vi "S4 Tool Initial.vi"(8 "error in (no error)":errorcluster) -> (0 "error constant":errorcluster, 3 "S4 InitialStatus":bool)   [LabVIEW 2019]
uses:
  Ctrl/StationCmdSelect.ctl
  Ctrl/Auto Inspection Station Name2.ctl
  Ctrl/Auto Inspection Data Name.ctl
  Global/Process Global.vi
  LineScan/LineScan.lvclass
  LLB/Commonly VI.lvlib
panel:
  out "ToolStringOut_Init":string
  out "Initial_ChkSum":string
  out "Initial receive 2":string
  in  "Numeric 3":i32
  out "Act Step":i32
  out "Numeric":dbl
  out "subarray":string[](array[string])
  out "retry次數":string[](array[string])
  out "CurrentCmd":string
  out "Retry":i32
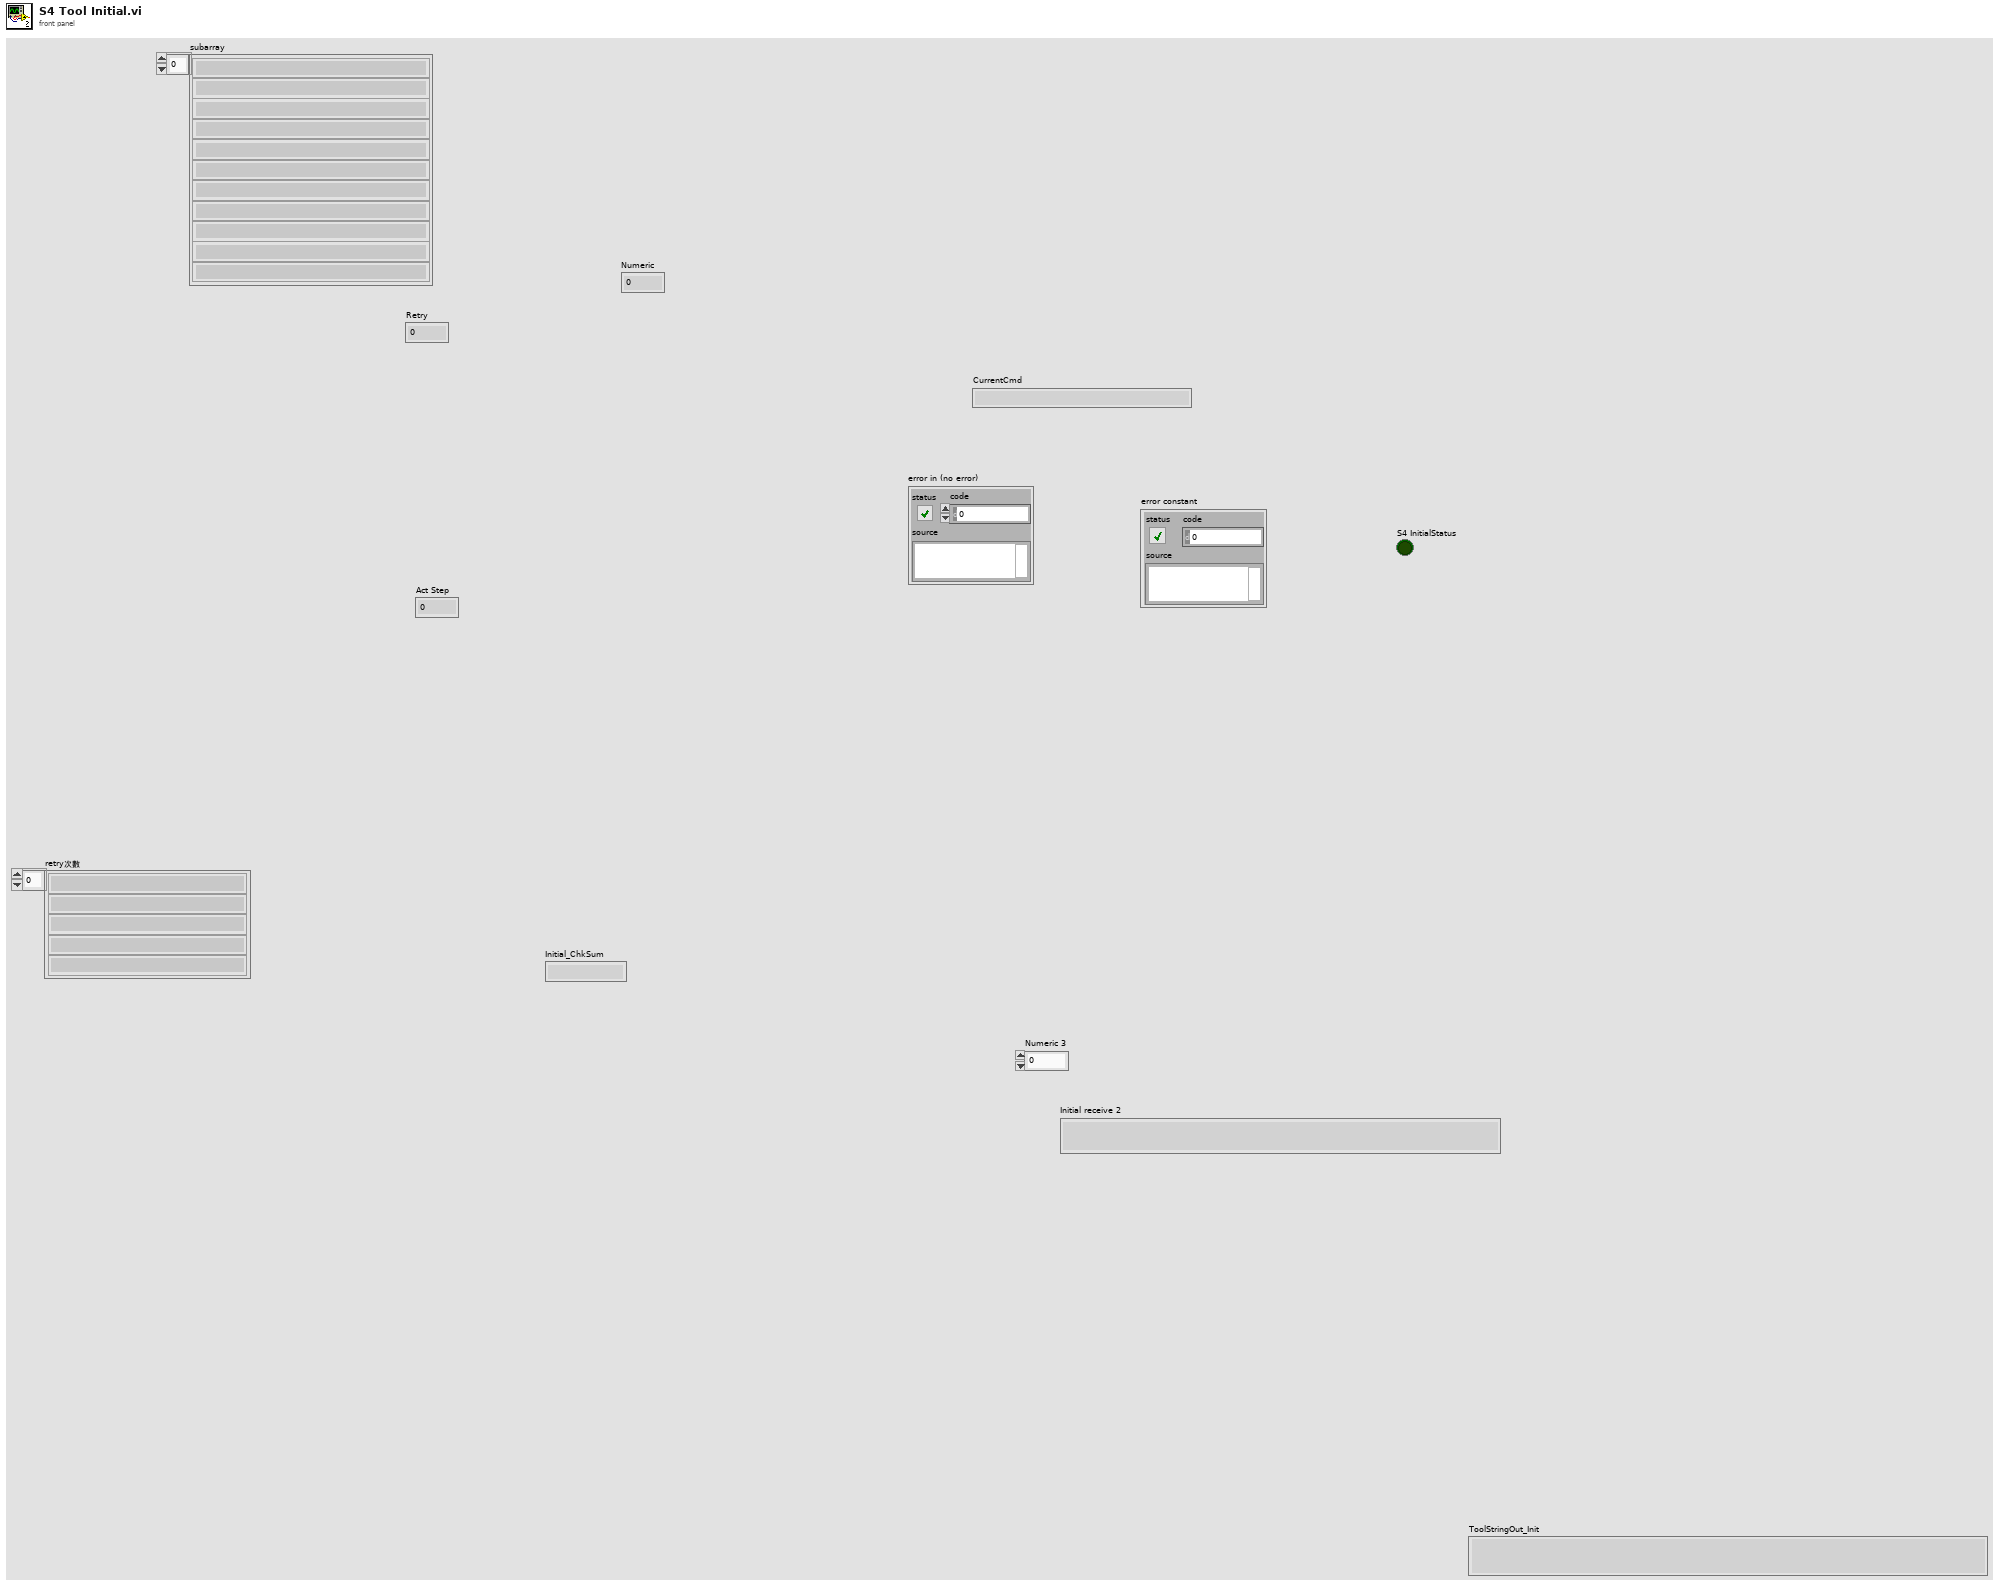
[diagram p1: front panel]
types:
  T1 = typedef "StationCmdSelect.ctl" = enum16{"Action", "Command", "Return", "DTime", "Retry"}
  T2 = typedef "Auto Inspection Data Name.ctl" = enum16{"LocalRun", "ItemSN(TimeCode)", "CurrentAction", "Error", "Data", "OKNG", "電壓值", "電壓值判斷", "電流值", "電流值判斷", "Laser1 Data", "Laser2 Data", "Laser OKNG", "StationNO"}
  T3 = typedef "Auto Inspection Station Name2.ctl" = enum16{"S1Barcode", "S2Measure", "S3Measure", "S4Measure", "S5Measure", "S11_LaserCheck", "S8_Vision AI"}
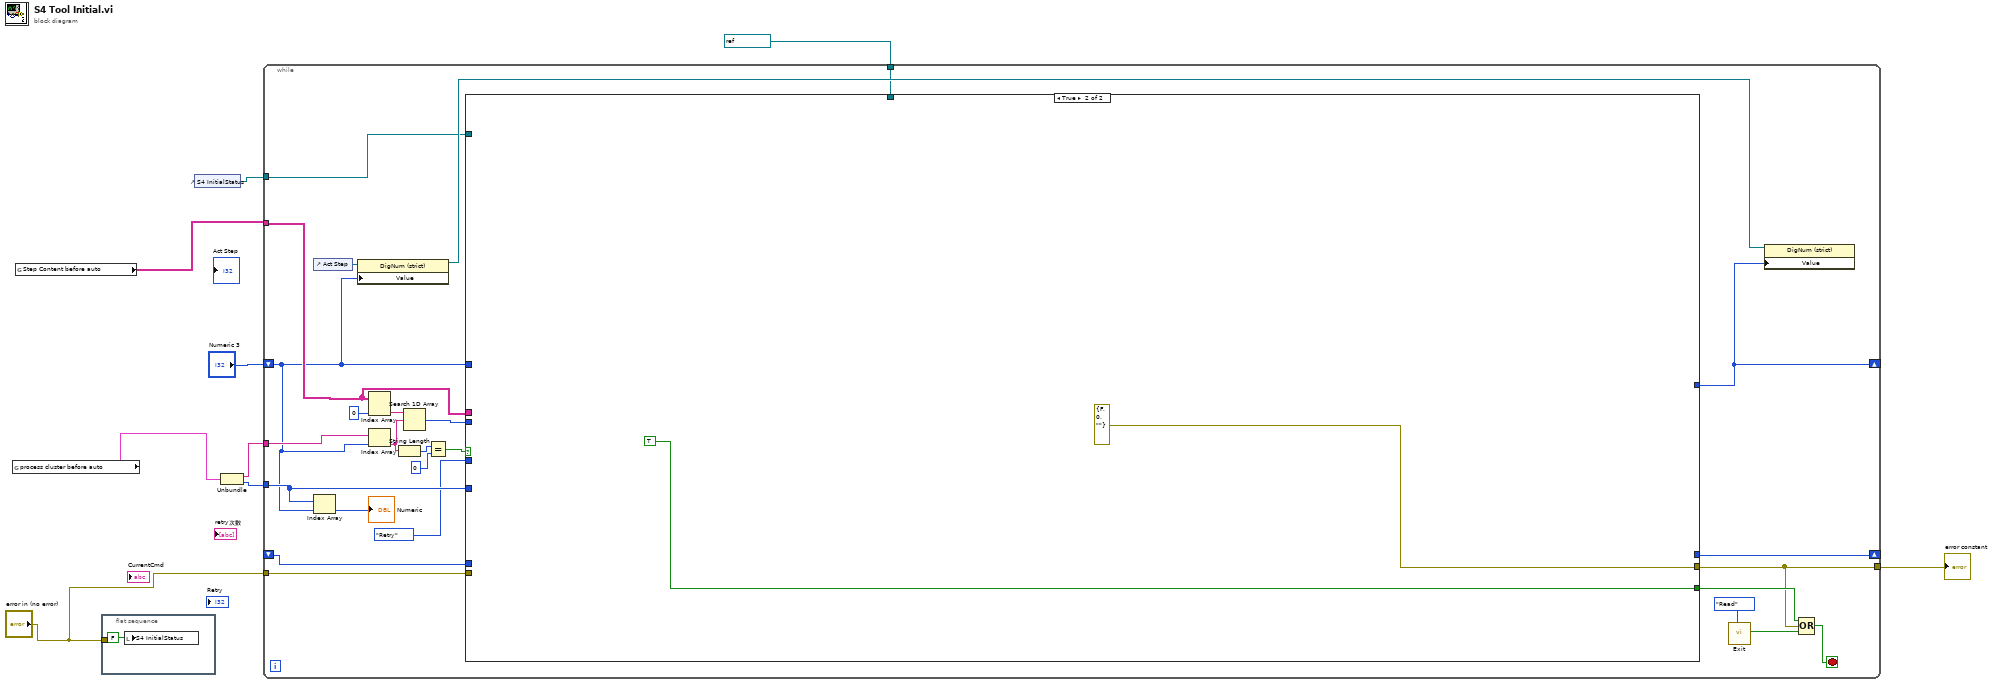
[diagram p0: block diagram]
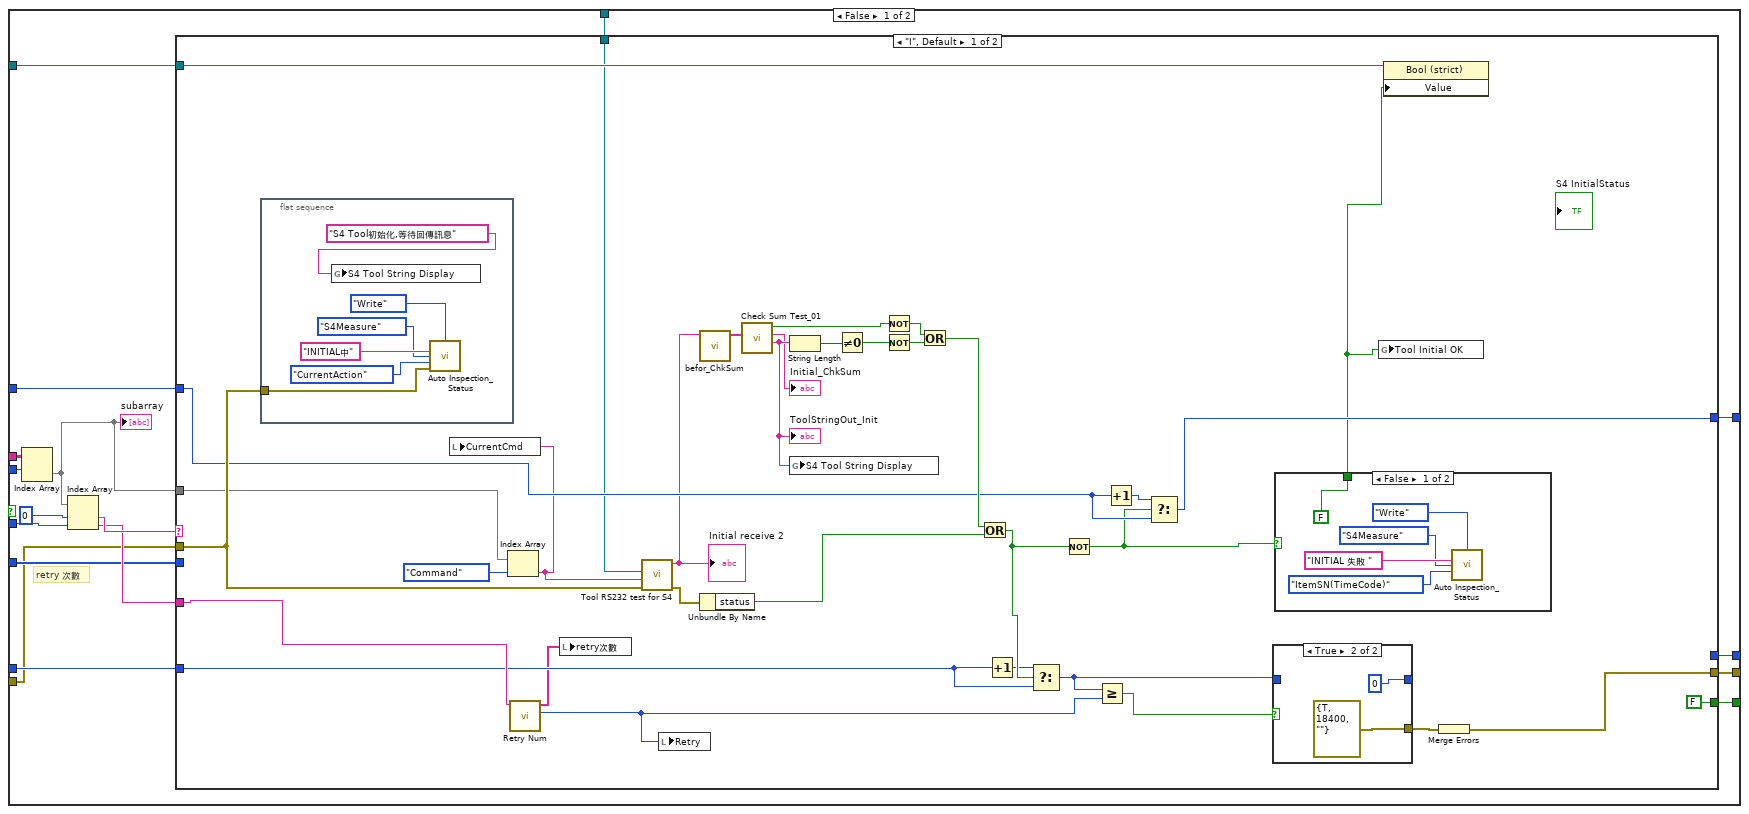
[diagram p2: hidden frame]
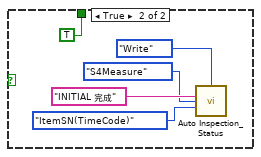
[diagram p3: hidden frame]
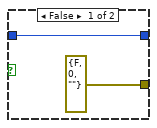
[diagram p4: hidden frame]
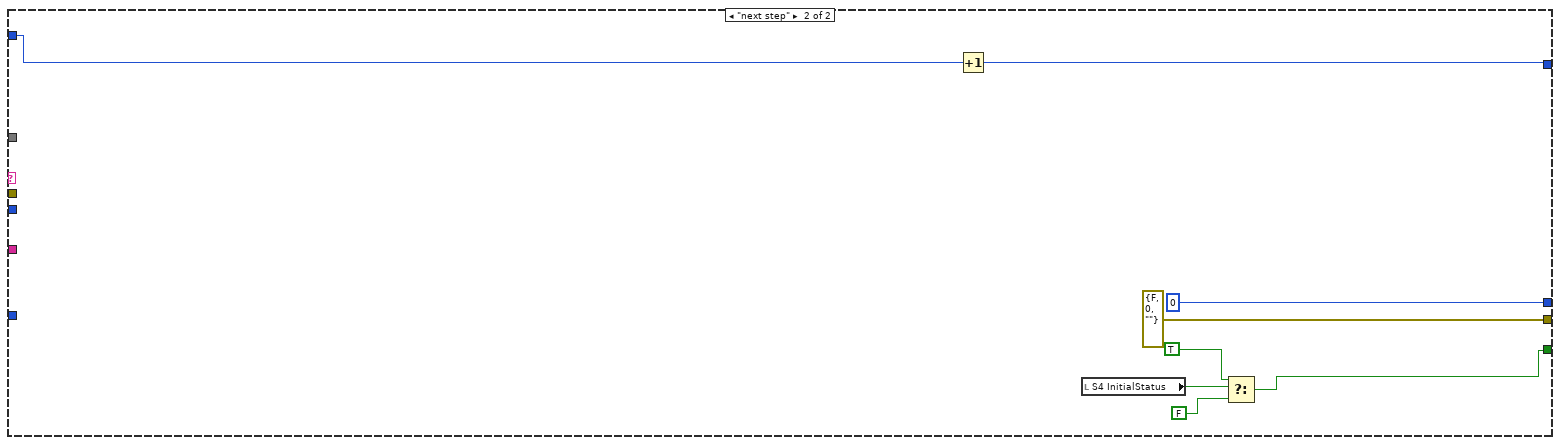
[diagram p5: hidden frame]
diagram:
  n1 = global read "Process Global.vi" "process cluster before auto"() -> (w4:cluster{string[], i32[]})
  n2 = global read "Process Global.vi" "Step Content before auto"() -> (w5:string[][])
  n3 = flat-sequence {
    tunnel: "error in (no error)" -> [_]
    frame #0 {
      n4 = local write "S4 InitialStatus"(FALSE ("S4 InitialStatus")) -> ()
    }
  }
  n5 = control-ref of="S4 InitialStatus"() -> (w3:refnum<vi>)
  n6 = Unbundle(w4) -> (w9:string[], w8:i32[])
  n7 = while {
    tunnel: w9 -> [w36]
    tunnel: w8 -> [w35]
    tunnel: w5 -> [w34]
    shift-right: [w19] -> _
    shift-left: _ -> [w23]
    shift-right: [w20] -> _
    shift-left: "Numeric 3" -> [w17]
    tunnel: [w16] -> w6
    tunnel: w3 -> [w15]
    tunnel: refnum<visa-resource-name> "COM2" ("VISA resource name") -> [w14]
    tunnel: "error in (no error)" -> [w11]
    stop <- w24 stop-if-true
    n8 = control-ref of="Act Step"() -> (w22:refnum<vi>)
    n9 = Index Array(array=w35, index=w17) -> (element=→"Numeric":i32)
    n10 = property class="DigNum (strict)"(reference=w22, "Value"=w17) -> (reference out=w21:refnum<vi>)  [unwired: 1 in, 1 out]
    n11 = Index Array(array=w34, index (col)=0 ("disabled index (col)")) -> (element=w32:string[])  [unwired: 1 in]
    n12 = Index Array(array=w36, index=w17) -> (element=w29:string)
    n13 = String Length(string=w29) -> (length=w28:i32)
    n14 = Search 1D Array(1D array=w32, element=w29) -> (index of element=w31:i32)  [unwired: 1 in]
    n15 = Equal?(x=w28, y=0) -> (x = y?=w26:bool)
    n16 = case shown="True" w26 {
      tunnel: w34 -> [w53 _]
      tunnel: w31 -> [w52 _]
      tunnel: w35 -> [w48 _]
      tunnel: w23 -> [w46 _]
      tunnel: StationCmdSelect."Retry" -> [w45 _]
      tunnel: [w44 errorcluster {"status"=FALSE, "code"=0, "source"=""} ("error constant")] -> w16
      tunnel: w17 -> [w43 _]
      tunnel: [w42 _] -> w20
      tunnel: [w41 _] -> w19
      tunnel: [w40 TRUE] -> w18
      tunnel: w15 -> [w39 _]
      tunnel: w14 -> [w38 _]
      tunnel: w11 -> [w37 _]
      frame False {
        # "retry 次數"
        n17 = Index Array(array=w53, index (row)=w52) -> (element=w47:string[])  [unwired: 1 in]
        "subarray" <- w47
        n18 = Index Array(array=w47, index #1=0 ("index"), index #2=w45) -> (element #1=w50:string, element #2=w49:string)
        n19 = case shown="\"I\", Default" w50 {
          tunnel: w48 -> [_ _]
          tunnel: w49 -> [w66 _]
          tunnel: w47 -> [w67 _]
          tunnel: w46 -> [w65 _]
          tunnel: [w58 errorcluster {"status"=FALSE, "code"=0, "source"=""} ("error constant")] -> w44
          tunnel: w43 -> [w64 w115]
          tunnel: [w57 w114] -> w42
          tunnel: [_ 0] -> w41
          tunnel: [FALSE w108] -> w40
          tunnel: w37 -> [w68 _]
          tunnel: w39 -> [w87 _]
          tunnel: w38 -> [w63 _]
          frame "I", Default {
            n20 = flat-sequence {
              tunnel: w68 -> [w89]
              frame #0 {
                n21 = global write "Process Global.vi" "S4 Tool String Display"("S4 Tool初始化,等待回傳訊息") -> ()
                n22 = call "Auto Inspection_Status.vi"("Action"=enum16{"Initial", "Write", "Read"}."Write", "DataIn"="INITIAL中", "Station"=Auto_Inspection_Station_Name2."S4Measure", "Data"=Auto_Inspection_Data_Name."CurrentAction", "error in"=w89) -> ()  [unwired: 8 in, 3 out]
              }
            }
            n23 = Index Array(array=w67, index=StationCmdSelect."Command") -> (element=w62:string)
            n24 = local write "CurrentCmd"(w62) -> ()
            n25 = call "Retry Num.vi"("String"=w66) -> ("Numeric"=w60:i32, "retry次數"=w61:string[])  [unwired: 9 in]
            n26 = local write "retry次數"(w61) -> ()
            n27 = call "Tool RS232 test for S4.vi"("error in (no error)"=w68, "Cmd In"=w62, "VISA resource name"=w63) -> ("error out"=w71:errorcluster, "receive string"=w55:string)  [unwired: 7 in]
            "Initial receive 2" <- w55
            n28 = local write "Retry"(w60) -> ()
            n29 = call "befor_ChkSum.vi"("ToolString Input"=w55) -> ("Array"=w81:string[])  [unwired: 9 in, 1 out]
            n30 = Unbundle By Name(w71) -> ("status"=w75:bool)
            n31 = call "Check Sum Test_01.vi"("Array"=w81) -> ("ToolStringOut_01"=w86:string, "ChkSum"=→"Initial_ChkSum":string, "x = y?"=w84:bool)  [unwired: 8 in]
            "ToolStringOut_Init" <- w86
            n32 = String Length(string=w86) -> (length=w78:i32)
            n33 = global write "Process Global.vi" "S4 Tool String Display"(w86) -> ()
            n34 = Not Equal To 0?(x=w78) -> (x != 0?=w77:bool)
            n35 = Not(x=w84) -> (.not. x?=w80:bool)
            n36 = Not(x=w77) -> (.not. x?=w79:bool)
            n37 = Or(x=w80, y=w79) -> (x .or. y?=w83:bool)
            n38 = Or(x=w83, y=w75) -> (x .or. y?=w76:bool)
            n39 = Increment(x=w65) -> (x+1=w70:i32)
            n40 = Select(t=w70, s=w76, f=w65) -> (s? t:f=w74:i32)
            n41 = Not(x=w76) -> (.not. x?=w59:bool)
            n42 = Greater Or Equal?(x=w74, y=w60) -> (x >= y?=w72:bool)
            n43 = Increment(x=w64) -> (x+1=w73:i32)
            n44 = Select(t=w73, s=w59, f=w64) -> (s? t:f=w57:i32)
            n45 = case shown="True" w72 {
              tunnel: [errorcluster {"status"=FALSE, "code"=0, "source"=""} ("error constant") errorcluster {"status"=TRUE, "code"=18400, "source"=""} ("error constant")] -> w85
              tunnel: w74 -> [w104 _]
              tunnel: [w104 0] -> _
              frame False {
              }
              frame True {
              }
            }
            n46 = case shown="False" w59 {
              tunnel: [FALSE TRUE] -> w54
              frame False {
                n47 = call "Auto Inspection_Status.vi"("Action"=enum16{"Initial", "Write", "Read"}."Write", "DataIn"="INITIAL 失敗 ", "Station"=Auto_Inspection_Station_Name2."S4Measure", "Data"=Auto_Inspection_Data_Name."ItemSN(TimeCode)") -> ()  [unwired: 9 in, 3 out]
              }
              frame True {
                n48 = call "Auto Inspection_Status.vi"("Action"=enum16{"Initial", "Write", "Read"}."Write", "DataIn"="INITIAL 完成", "Station"=Auto_Inspection_Station_Name2."S4Measure", "Data"=Auto_Inspection_Data_Name."ItemSN(TimeCode)") -> ()  [unwired: 9 in, 3 out]
              }
            }
            n49 = global write "Process Global.vi" "Tool Initial OK"(w54) -> ()
            n50 = property class="Bool (strict)"(reference=w87, "Value"=w54) -> ()  [unwired: 1 in, 2 out]
            n51 = Merge Errors(w85) -> (w58:errorcluster)
          }
          frame "next step" {
            n52 = Increment(x=w115) -> (x+1=w114:i32)
            n53 = local read "S4 InitialStatus"() -> (w110:bool)
            n54 = Select(t=TRUE, s=w110, f=FALSE) -> (s? t:f=w108:bool)
          }
        }
      }
      frame True {
      }
    }
    n55 = call "Exit.vi"("Enum"=enum16{"Initial", "Read", "Write"}."Read") -> ("ExitOut"=w12:bool)  [unwired: 10 in]
    n56 = property class="DigNum (strict)"(reference=w21, "Value"=w20) -> ()  [unwired: 1 in, 2 out]
    n57 = Compound Arithmetic op=OR(w18, w16, w12) -> (w24:bool)
  }
  "error constant" <- w6
